vi "ExWriteFileTypes.vi"() -> ()   [LabVIEW 2010]
panel:
  out "error out":errorcluster
  in  "error in (no error)":errorcluster
  out "String":string
  in  "Y Size":u32=1 min=1 step=1
  in  "X Size":u32=1 min=1 step=1
  in  "File Name":path
  in  "Data Type":u16(ring)=6 items=["", "8 Bit Unsigned Integer", "16 Bit Unsigned Integer", "32 Bit Unsigned Integer", "32 Bit Floating Point"]
  in  "File Type":u16(ring)=1 items=["PMI (Photometrics)", "SPE (Princeton Instruments)", "TIFF"]
  # "ExWriteFileTypes.vi\nThis Example will create a new file of the\ntype specified and fill it with demo data of\nthe form p(x,y) = (y*100) + x"
  # "NOTICE\n\nTHIS VI REQUIRES THAT THE TOOLKIT\nBE UNLOADED BY RUNNING THE\n VI EXCLOSEGLOBALCAM.VI\n BEFORE LEAVING LABVIEW."
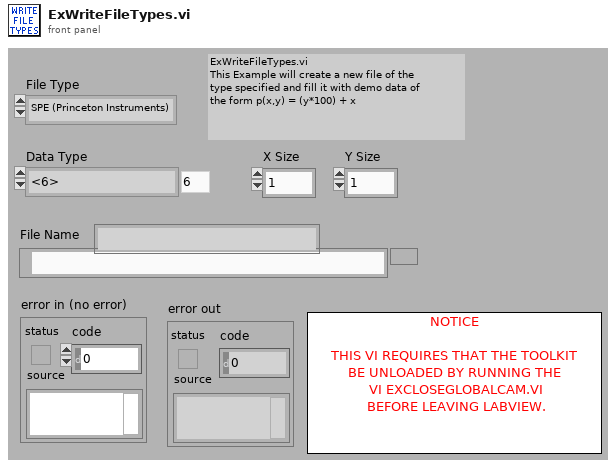
[diagram p1: front panel]
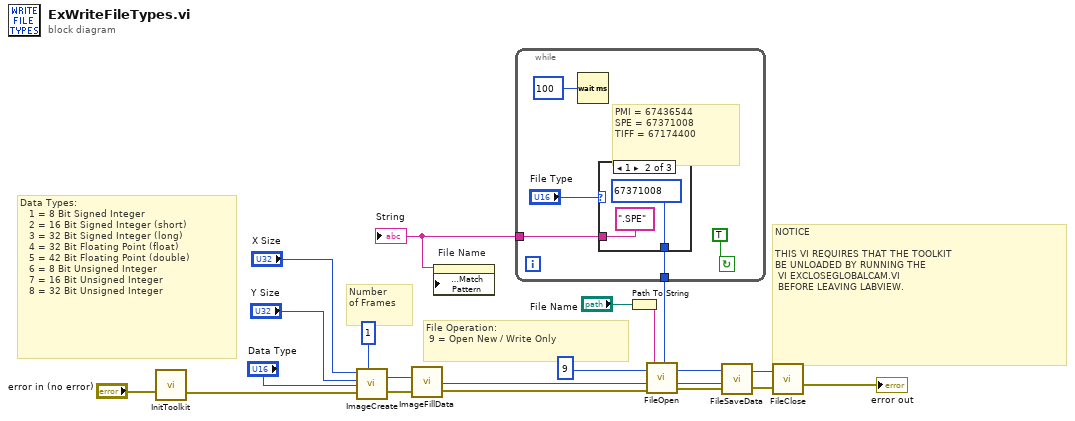
[diagram p0: block diagram]
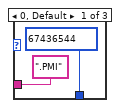
[diagram p2: hidden frame]
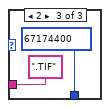
[diagram p3: hidden frame]
diagram:
  # "NOTICE\n\nTHIS VI REQUIRES THAT THE TOOLKIT\nBE UNLOADED BY RUNNING THE\n VI EXCLOSEGLOBALCAM.VI\n BEFORE LEAVING LABVIEW."
  # "Data Types:\n   1 = 8 Bit Signed Integer\n   2 = 16 Bit Signed Integer (short)\n   3 = 32 Bit Signed Integer (long)\n   4 = 32 Bit Floating Point (float)\n   5 = 42 Bit Floating Point (double)\n   6 = 8 Bit Unsigned Integer\n   7 = 16 Bit Unsigned Integer\n   8 = 32 Bit Unsigned Integer"
  # "Number\nof Frames"
  # "File Operation:\n 9 = Open New / Write Only"
  n1 = call <userlib>:"InitToolkit.vi"("error in"="error in (no error)") -> ("error out"=w16:errorcluster)
  n2 = call <userlib>:"ImageCreate.vi"("X dimension"="X Size", "Y dimension"="Y Size", "Data Type"="Data Type", "error in"=w16, "Number Of Frames"=1) -> ("Image Handle"=w19:u32, "error out"=w20:errorcluster)
  n3 = call <userlib>:"ImageFillData.vi"("error in"=w20, "Image Handle"=w19) -> ("error out"=w8:errorcluster, "Image Handle"=w15:u32)  [unwired: 1 in]
  n4 = while {
    tunnel: [w24] -> w5
    tunnel: [w23] -> w3
    stop <- TRUE continue-if-true
    # "PMI = 67436544\nSPE = 67371008\nTIFF = 67174400"
    n5 = Wait (ms)(milliseconds to wait=100) -> ()  [unwired: 1 out]
    n6 = case shown="1" "File Type" {
      tunnel: [67436544 67371008 67174400] -> w23
      tunnel: [".PMI" ("String") ".SPE" ("String") ".TIF" ("String")] -> w24
      frame 0, Default {
      }
      frame 1 {
      }
      frame 2 {
      }
    }
  }
  "String" <- w5
  n7 = property on="File Name" class="Path"("Browse Options:Match Pattern"=w5) -> ()  [unwired: 2 in, 2 out]
  n8 = Path To String(path="File Name") -> (string=w10:string)
  n9 = call <userlib>:"FileOpen.vi"("error in"=w8, "File Operations"=9, "FileName"=w10, "File Type"=w3) -> ("error out"=w7:errorcluster, "File Handle"=w4:u32)
  n10 = call <userlib>:"FileSaveData.vi"("error in"=w7, "Image Handle"=w15, "File Handle"=w4) -> ("error out"=w17:errorcluster, "File Handle"=w14:u32)
  n11 = call <userlib>:"FileClose.vi"("error in"=w17, "File Handle"=w14) -> ("error out"=→"error out":errorcluster)
